vi "display_1s_stim_9s_ISI_CS1_CS2_blocks_no_trigger.vi"() -> ()   [LabVIEW 2019]
uses:
  <vilib>/Analysis/Matrix/Datatypes/RealMatrix.ctl
  <vilib>/Utility/file.llb/Write Delimited Spreadsheet (DBL).vi
  <vilib>/Analysis/Matrix/NI_Matrix.lvlib
panel:
  out "ISI Time":dbl
  out "Stim TS":dbl
  out "Output":dbl[][](array[numeric])
  out "Output frame":T1
  out "Frame_clock":u32
  out "Array temp1":T1
  out "Elapsed Time":dbl
  out "Display":bool=TRUE
  out "Trial":u32=1
  out "reward":dbl[](array[numeric])
  out "stim_id":dbl[](array[numeric])
  out "stim_loaded":dbl
  out "Timings":dbl[](array[numeric])
  out "Stimuli Loaded?":bool
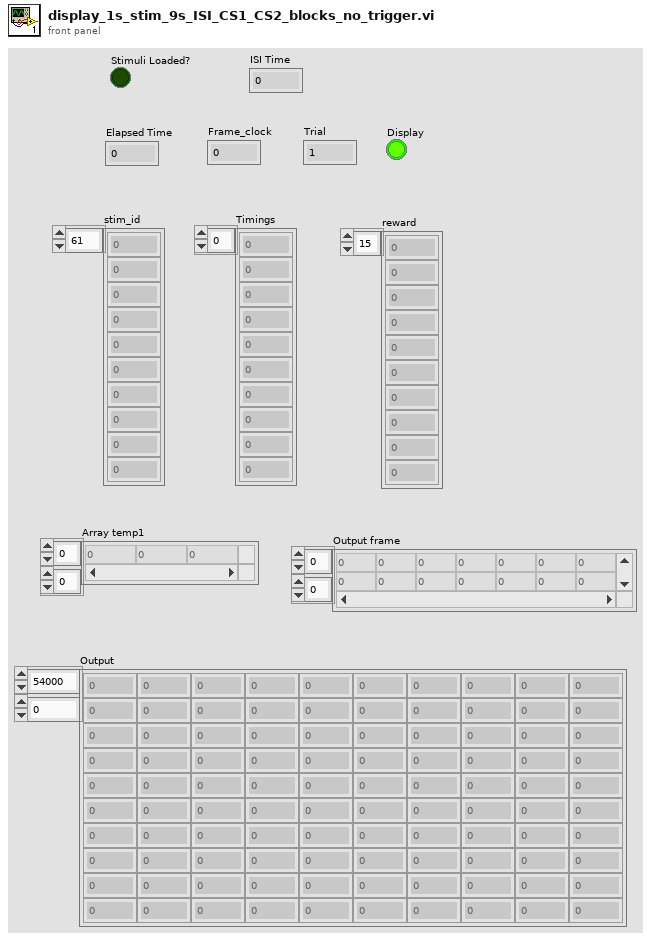
[diagram p1: front panel]
types:
  T1 = typedef "NI_Matrix.lvlib/RealMatrix.ctl" = dbl[][]
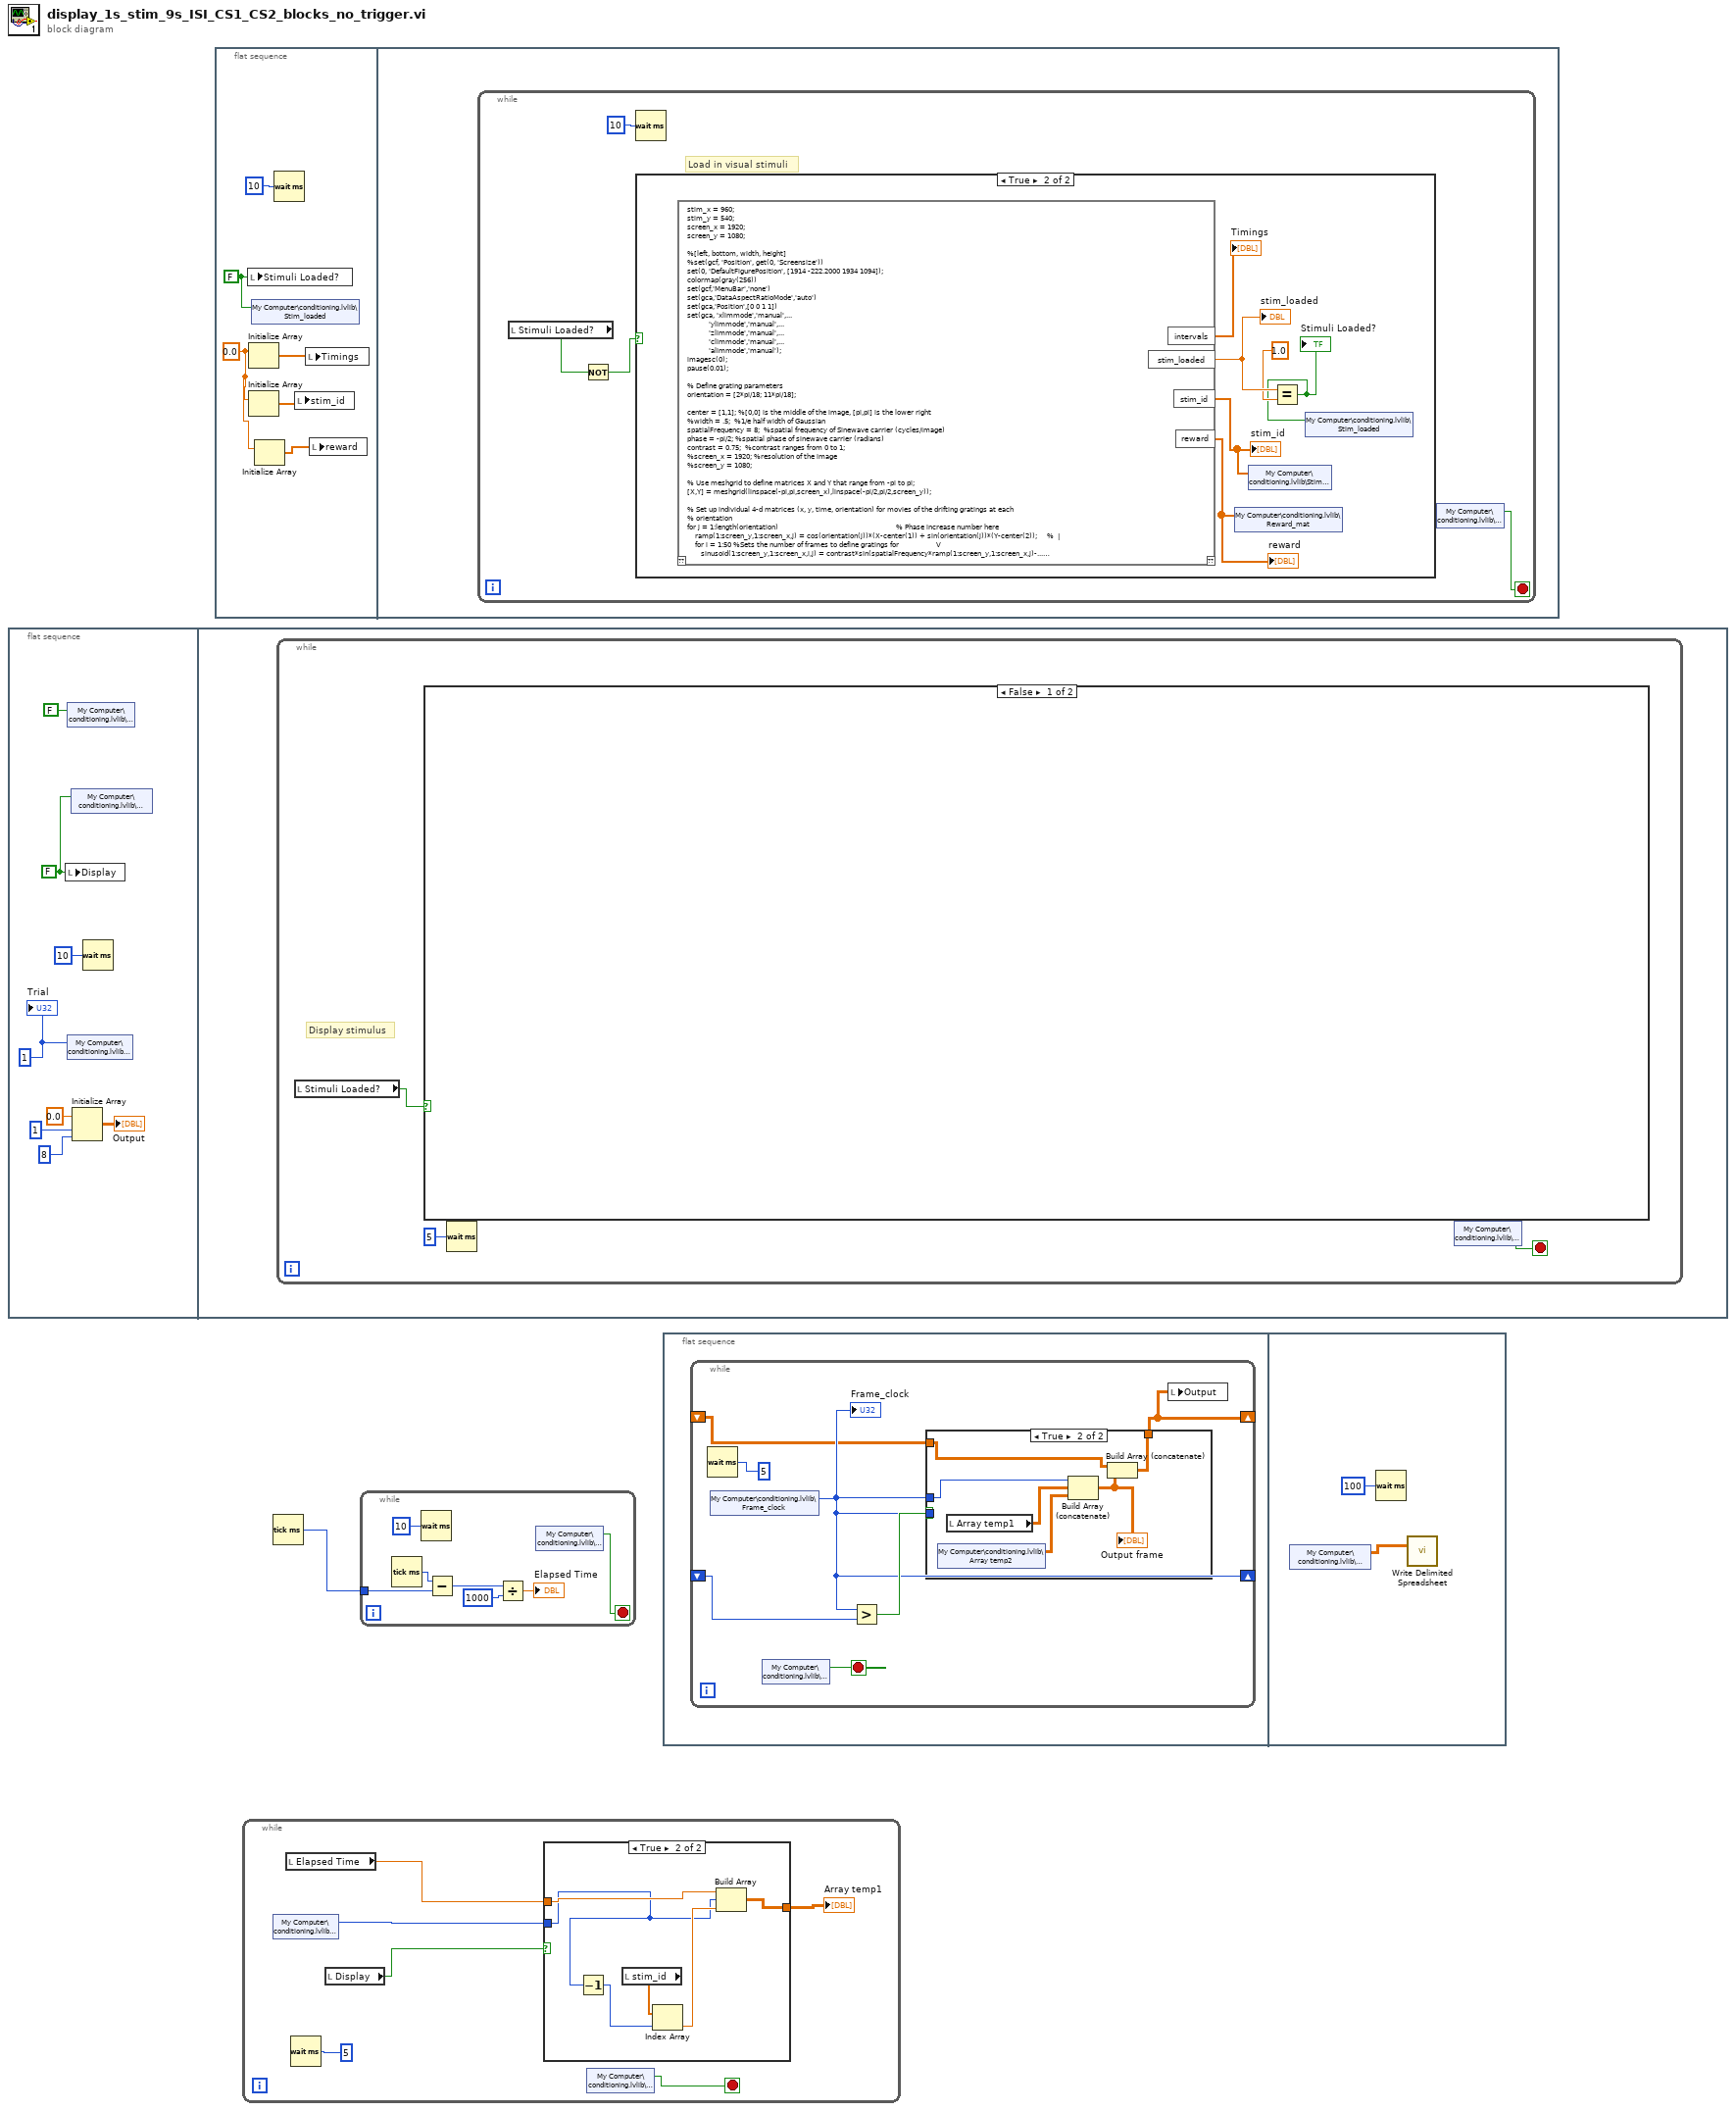
[diagram p0: block diagram]
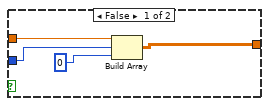
[diagram p2: hidden frame]
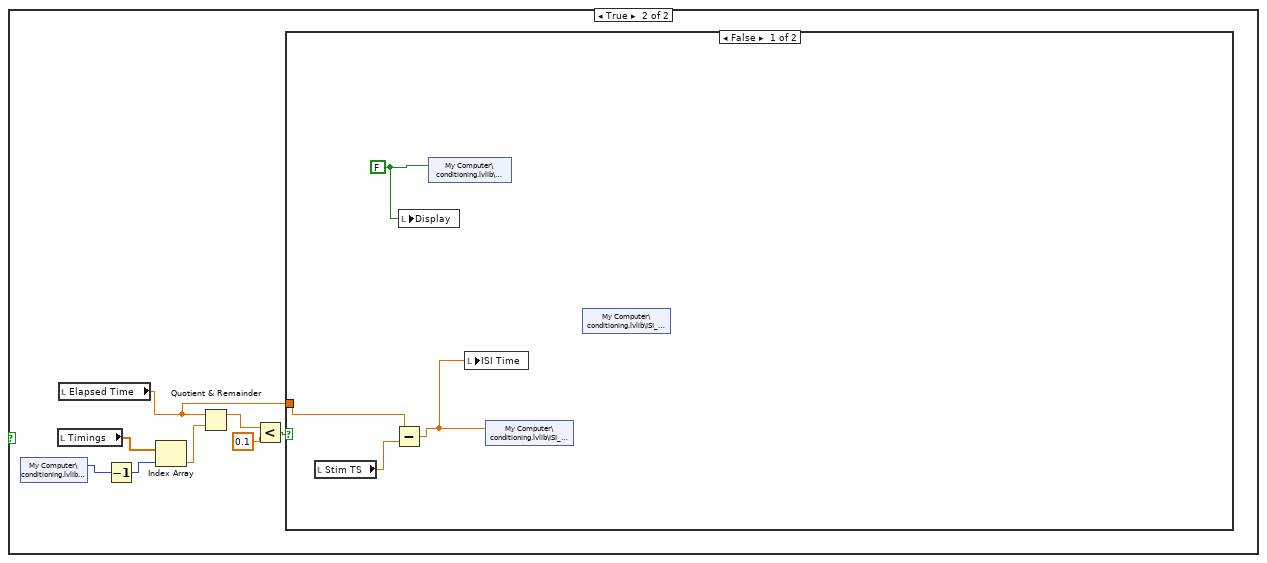
[diagram p5: hidden frame]
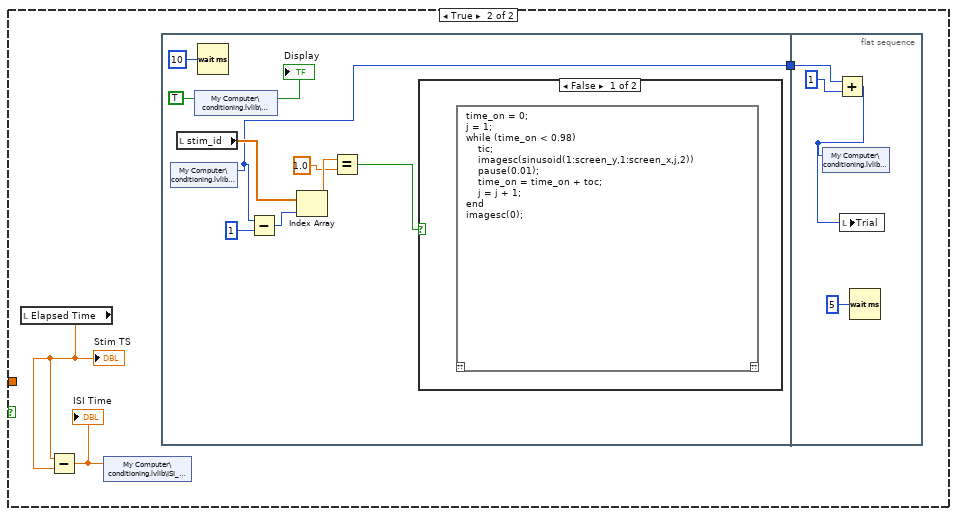
[diagram p6: hidden frame]
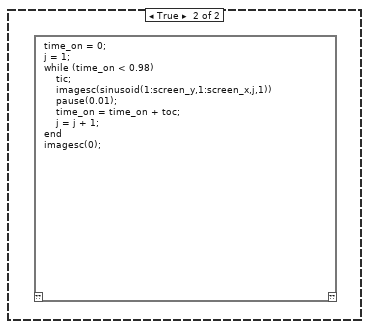
[diagram p7: hidden frame]
diagram:
  n1 = flat-sequence {
    frame #0 {
      w7 = FALSE ("Display")
      w9 = u32 1 ("Trial")
      n2 = local write "Display"(w7) -> ()
      n3 = shared-variable "My Computer\\conditioning.lvlib\\Stop"(FALSE ("Stop")) -> ()  [unwired: 1 in, 1 out]
      n4 = shared-variable "My Computer\\conditioning.lvlib\\Trial"(w9) -> ()  [unwired: 1 in, 1 out]
      n5 = shared-variable "My Computer\\conditioning.lvlib\\Display"(w7) -> ()  [unwired: 1 in, 1 out]
      n6 = Initialize Array(0.0 ("element"), 1 ("dimension size"), 8 ("dimension size")) -> (→"Output":dbl[][])
      n7 = Wait (ms)(milliseconds to wait=u32 10) -> ()  [unwired: 1 out]
      "Trial" <- w9
    }
    frame #1 {
      n8 = while {
        stop <- w11 stop-if-true
        # "Display stimulus"
        n9 = local read "Stimuli Loaded?"() -> (w10:bool)
        n10 = case shown="False" w10 {
          frame False {
          }
          frame True {
            n11 = shared-variable "My Computer\\conditioning.lvlib\\Trial"() -> (w16:u32)  [unwired: 1 in, 1 out]
            n12 = local read "Timings"() -> (w17:dbl[])
            n13 = local read "Elapsed Time"() -> (w13:dbl)
            n14 = Decrement(x=w16) -> (x-1=w15:u32)
            n15 = Index Array(array=w17, index=w15) -> (element=w14:dbl)
            n16 = Quotient & Remainder(x=w13, y=w14) -> (x-y*floor(x/y)=w20:dbl)  [unwired: 1 out]
            n17 = Less?(x=w20, y=0.1) -> (x < y?=w18:bool)
            n18 = case shown="False" w18 {
              tunnel: w13 -> [w23 _]
              frame False {
                w24 = FALSE ("Display")
                n19 = local read "Stim TS"() -> (w22:dbl)
                n20 = Subtract(x=w23, y=w22) -> (x-y=w21:dbl)
                n21 = local write "Display"(w24) -> ()
                n22 = shared-variable "My Computer\\conditioning.lvlib\\Display"(w24) -> ()  [unwired: 1 in, 1 out]
                n23 = local write "ISI Time"(w21) -> ()
                n24 = shared-variable "My Computer\\conditioning.lvlib\\ISI_Time"(w21) -> ()  [unwired: 1 in, 1 out]
                n25 = shared-variable "My Computer\\conditioning.lvlib\\ISI_Time"() -> ()  [unwired: 1 in, 2 out]
              }
              frame True {
                n26 = local read "Elapsed Time"() -> (w26:dbl)
                "Stim TS" <- w26
                n27 = Subtract(x=w26, y=w26) -> (x-y=w25:dbl)
                "ISI Time" <- w25
                n28 = shared-variable "My Computer\\conditioning.lvlib\\ISI_Time"(w25) -> ()  [unwired: 1 in, 1 out]
                n29 = flat-sequence {
                  tunnel: [w30] -> w27
                  tunnel: w27 -> [w40]
                  frame #0 {
                    w32 = TRUE ("Boolean")
                    n30 = shared-variable "My Computer\\conditioning.lvlib\\Trial"() -> (w30:u32)  [unwired: 1 in, 1 out]
                    n31 = local read "stim_id"() -> (w35:dbl[])
                    n32 = shared-variable "My Computer\\conditioning.lvlib\\Display"(w32) -> ()  [unwired: 1 in, 1 out]
                    n33 = Wait (ms)(milliseconds to wait=u32 10) -> ()  [unwired: 1 out]
                    n34 = Subtract(x=w30, y=u32 1) -> (x-y=w31:u32)
                    n35 = Index Array(array=w35, index=w31) -> (element=w34:dbl)
                    n36 = Equal?(x=w34, y=1.0) -> (x = y?=w28:bool)
                    n37 = case shown="False" w28 {
                      frame False {
                        n38 = script code="time_on = 0;\nj = 1;\nwhile (time_on < 0.98)\n    tic;\n    imagesc(sinusoid(1:screen_y,1:screen_x,j,2))\n    pause(0.01);\n    time_on = time_on + toc;\n    j = j + 1;\nend\nimagesc(0);"() -> ()  [unwired: 1 in, 1 out]
                      }
                      frame True {
                        n39 = script code="time_on = 0;\nj = 1;\nwhile (time_on < 0.98)\n    tic;\n    imagesc(sinusoid(1:screen_y,1:screen_x,j,1))\n    pause(0.01);\n    time_on = time_on + toc;\n    j = j + 1;\nend\nimagesc(0);"() -> ()  [unwired: 1 in, 1 out]
                      }
                    }
                    "Display" <- w32
                  }
                  frame #1 {
                    n40 = Add(x=w40, y=u32 1) -> (x+y=w38:u32)
                    n41 = shared-variable "My Computer\\conditioning.lvlib\\Trial"(w38) -> ()  [unwired: 1 in, 1 out]
                    n42 = local write "Trial"(w38) -> ()
                    n43 = Wait (ms)(milliseconds to wait=u32 5) -> ()  [unwired: 1 out]
                  }
                }
              }
            }
          }
        }
        n44 = Wait (ms)(milliseconds to wait=u32 5) -> ()  [unwired: 1 out]
        n45 = shared-variable "My Computer\\conditioning.lvlib\\Stop"() -> (w11:bool)  [unwired: 1 in, 1 out]
      }
    }
  }
  n46 = flat-sequence {
    frame #0 {
      w43 = 0.0 ("element")
      w41 = FALSE ("Stimuli Loaded?")
      n47 = local write "Stimuli Loaded?"(w41) -> ()
      n48 = Initialize Array(w43) -> (w45:dbl[])  [unwired: 1 in]
      n49 = Initialize Array(w43) -> (w44:dbl[])  [unwired: 1 in]
      n50 = shared-variable "My Computer\\conditioning.lvlib\\Stim_loaded"(w41) -> ()  [unwired: 1 in, 1 out]
      n51 = Initialize Array(w43) -> (w42:dbl[])  [unwired: 1 in]
      n52 = Wait (ms)(milliseconds to wait=u32 10) -> ()  [unwired: 1 out]
      n53 = local write "stim_id"(w44) -> ()
      n54 = local write "Timings"(w45) -> ()
      n55 = local write "reward"(w42) -> ()
    }
    frame #1 {
      n56 = while {
        stop <- w49 stop-if-true
        # "Load in visual stimuli"
        n57 = local read "Stimuli Loaded?"() -> (w48:bool)
        n58 = Not(x=w48) -> (.not. x?=w47:bool)
        n59 = Wait (ms)(milliseconds to wait=u32 10) -> ()  [unwired: 1 out]
        n60 = case shown="True" w47 {
          frame False {
          }
          frame True {
            n61 = script code="stim_x = 960;\nstim_y = 540;\nscreen_x = 1920;\nscreen_y = 1080;\n\n%[left, bottom, width, height]\n%set(gcf, 'Position', get(0, 'Screensize'))\nset(0, 'DefaultFigurePosition', [1914 -222.2000 1934 1094]);\ncolormap(gray(256))\nset(gcf,'MenuBar','none')\nset(gca,'DataAspectRatioMode','auto')\nset(gca,'Position',[0 0 1 1])\nset(gca, 'xlimmode','manual',...\n           'ylimmode','manual',...\n           'zlimmode','manual',...\n           'climmode','manual',...\n           'alimmode','manual');\nimagesc(0);\npause(0.01);\n\n% Define grating parameters\norientation = [2*pi/18; 11*pi/18];\n\ncenter = [1,1]; %[0,0] is the middle of the image, [pi,pi] is the lower right\n%width = .5;  %1/e half width of Gaussian\nspatialFrequency = 8;  %spatial frequency of Sinewave carrier (cycles/image)\nphase = -pi/2; %spatial phase of sinewave carrier (radians)\ncontrast = 0.75;  %contrast ranges from 0 to 1;\n%screen_x = 1920; %resolution of the image  \n%screen_y = 1080;\n\n% Use meshgrid to define matrices X and Y that range from -pi to pi;\n[X,Y] = meshgrid(linspace(-pi,pi,screen_x),linspace(-pi/2,pi/2,screen_y));\n\n% Set up individual 4-d matrices (x, y, time, orientation) for movies of the drifting gratings at each\n% orientation\nfor j = 1:length(orientation)                                                            % Phase increase number here\n    ramp(1:screen_y,1:screen_x,j) = cos(orientation(j))*(X-center(1)) + sin(orientation(j))*(Y-center(2));     %  |\n    for i = 1:50 %Sets the number of frames to define gratings for                   V\n       sinusoid(1:screen_y,1:screen_x,i,j) = contrast*sin(spatialFrequency*ramp(1:screen_y,1:screen_x,j)-...\n           (phase+(2*pi*(i-1)*(-30)/360))); %Number before '/360' sets the phase increase\n    end\nend\n\nintervals = [ones(1,204)*12];\nstim_id = [ones(1,34)*1 ones(1,34)*2 ones(1,34)*1 ones(1,34)*2 ones(1,34)*1 ones(1,34)*2];\nreward = [ones(1,204)];\n\nstim_loaded = 1;" ("Script Node")() -> ("stim_loaded"=w56:dbl, "intervals"=→"Timings":dbl[], "stim_id"=w51:dbl[], "reward"=w53:dbl[])  [unwired: 1 in, 1 out]
            "stim_loaded" <- w56
            "stim_id" <- w51
            "reward" <- w53
            n62 = shared-variable "My Computer\\conditioning.lvlib\\Reward_mat"(w53) -> ()  [unwired: 1 in, 1 out]
            n63 = shared-variable "My Computer\\conditioning.lvlib\\Stim_ID"(w51) -> ()  [unwired: 1 in, 1 out]
            n64 = Equal?(x=w56, y=1.0) -> (x = y?=w52:bool)
            "Stimuli Loaded?" <- w52
            n65 = shared-variable "My Computer\\conditioning.lvlib\\Stim_loaded"(w52) -> ()  [unwired: 1 in, 1 out]
          }
        }
        n66 = shared-variable "My Computer\\conditioning.lvlib\\Stop"() -> (w49:bool)  [unwired: 1 in, 1 out]
      }
    }
  }
  n67 = while {
    stop <- w57 stop-if-true
    n68 = shared-variable "My Computer\\conditioning.lvlib\\Trial"() -> (w59:u32)  [unwired: 1 in, 1 out]
    n69 = local read "Elapsed Time"() -> (w61:dbl)
    n70 = Wait (ms)(milliseconds to wait=u32 5) -> ()  [unwired: 1 out]
    n71 = local read "Display"() -> (w58:bool)
    n72 = case shown="True" w58 {
      tunnel: w59 -> [w65 w68]
      tunnel: w61 -> [w66 w70]
      tunnel: [w64 w71] -> w60
      frame False {
        n73 = Build Array(w66, w65, u32 0 ("milliseconds to wait")) -> (w64:T1)
      }
      frame True {
        n74 = Decrement(x=w68) -> (x-1=w67:u32)
        n75 = local read "stim_id"() -> (w72:dbl[])
        n76 = Index Array(array=w72, index=w67) -> (element=w69:dbl)
        n77 = Build Array(w70, w68, w69) -> (w71:T1)
      }
    }
    "Array temp1" <- w60
    n78 = shared-variable "My Computer\\conditioning.lvlib\\Stop"() -> (w57:bool)  [unwired: 1 in, 1 out]
  }
  n79 = Tick Count (ms)() -> (millisecond timer value=w1:u32)
  n80 = while {
    tunnel: w1 -> [w76]
    stop <- w73 stop-if-true
    n81 = Tick Count (ms)() -> (millisecond timer value=w77:u32)
    n82 = Wait (ms)(milliseconds to wait=u32 10) -> ()  [unwired: 1 out]
    n83 = Subtract(x=w77, y=w76) -> (x-y=w74:u32)
    n84 = Divide(x=w74, y=u32 1000) -> (x/y=→"Elapsed Time":dbl)
    n85 = shared-variable "My Computer\\conditioning.lvlib\\Stop"() -> (w73:bool)  [unwired: 1 in, 1 out]
  }
  n86 = flat-sequence {
    frame #0 {
      n87 = while {
        shift-right: [w82] -> _
        shift-left: _ -> [w84]
        shift-right: [w80] -> _
        shift-left: _ -> [w81]
        stop <- w86 stop-if-true
        n88 = Wait (ms)(milliseconds to wait=u32 5) -> ()  [unwired: 1 out]
        n89 = shared-variable "My Computer\\conditioning.lvlib\\Frame_clock"() -> (w82:u32)  [unwired: 1 in, 1 out]
        "Frame_clock" <- w82
        n90 = shared-variable "My Computer\\conditioning.lvlib\\Stop"() -> (w86:bool)  [unwired: 1 in, 1 out]
        n91 = Greater?(x=w82, y=w84) -> (0:w83:bool)
        n92 = case shown="True" w83 {
          tunnel: w82 -> [_ _]
          tunnel: w82 -> [_ w93]
          tunnel: [w87 w89] -> w80
          tunnel: w81 -> [w87 w88]
          frame False {
          }
          frame True {
            n93 = shared-variable "My Computer\\conditioning.lvlib\\Array temp2"() -> (w91:dbl[][])  [unwired: 1 in, 1 out]
            n94 = local read "Array temp1"() -> (w92:T1)
            n95 = Build Array (concatenate)(w93, w92, w91) -> (w90:T1)
            "Output frame" <- w90
            n96 = Build Array (concatenate) ("Build Matrix")(w88, w90) -> (w89:T1)
          }
        }
        n97 = local write "Output"(w80) -> ()
      }
    }
    frame #1 {
      n98 = shared-variable "My Computer\\conditioning.lvlib\\Output"() -> (w95:dbl[][])  [unwired: 1 in, 1 out]
      n99 = Wait (ms)(milliseconds to wait=u32 100) -> ()  [unwired: 1 out]
      n100 = call-poly <vilib>:"Write Delimited Spreadsheet.vi"("2D data"=w95) -> ()  [unwired: 13 in, 2 out]
    }
  }
